vi "查询clonm对应的所有内容.vi"(7 "条件":enum16{"DISTINCT", "MIN", "MAX"}(ring), 8 "error in (no error)":errorcluster caption="错误输入（无错误）", 9 "组合框":string(combo), 10 "database":string="database1.mdb", 11 "table":string(combo)="CODMn") -> (0 "error out":errorcluster caption="错误输出", 3 "输出数组":string[](array[string]))   [LabVIEW 2016]
uses:
  <vilib>/addons/database/Connection.llb/DB Tools Open Connec (String).vi
  <vilib>/addons/database/Connection.llb/Conn Execute.vi
  <vilib>/addons/database/Recordset.llb/Rec Fetch Recordset Data (R).vi
  <vilib>/addons/database/Recordset.llb/Rec Destroy - Connection.vi
  <vilib>/addons/database/_DB Variant To Data/Database Variant To Data.xnode
  <vilib>/addons/database/NI_Database_API.lvlib
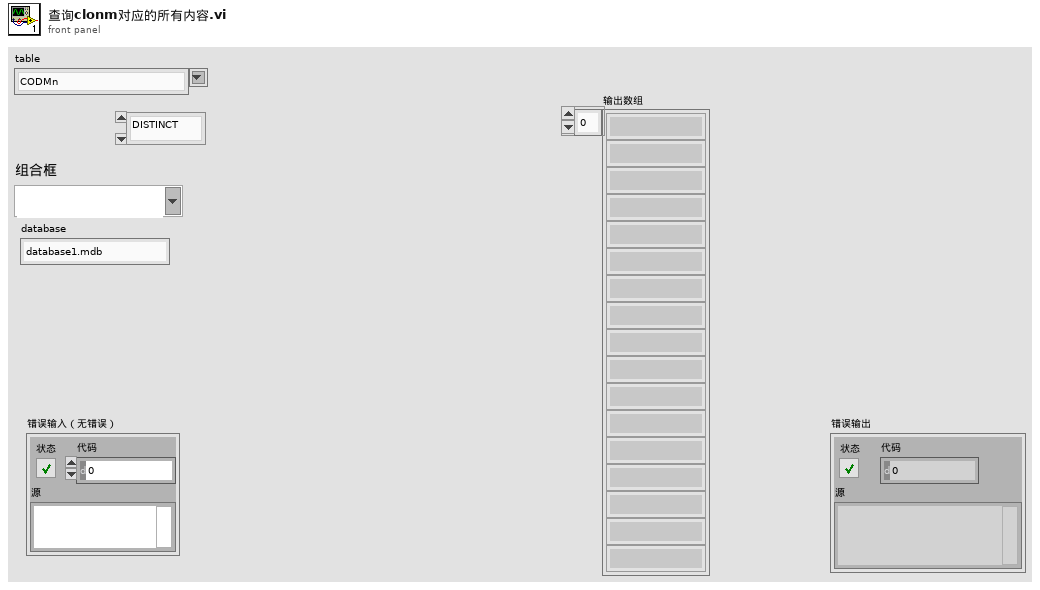
[diagram p1: front panel]
types:
  T1 = typedef "NI_Database_API.lvlib/Conn ObjectReference.ctl" = refnum<k1>
  T2 = typedef "NI_Database_API.lvlib/Rec ObjectReference.ctl" = refnum<k1>
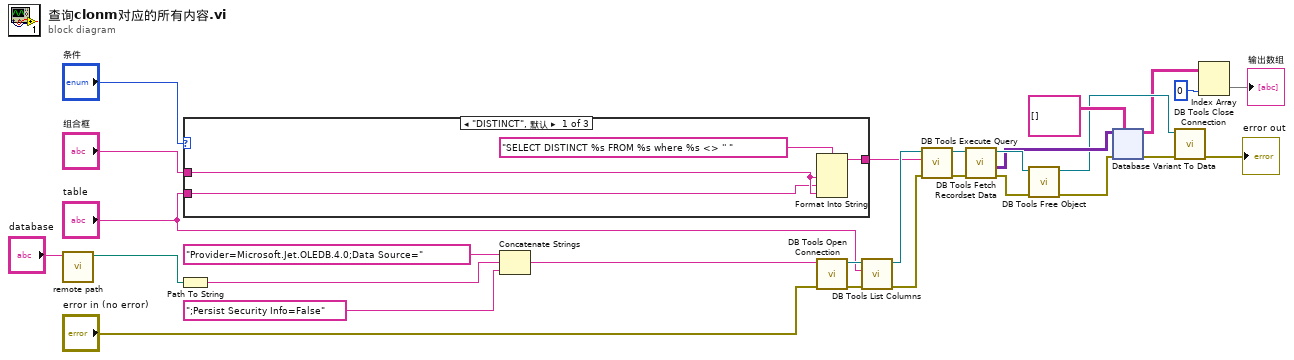
[diagram p0: block diagram]
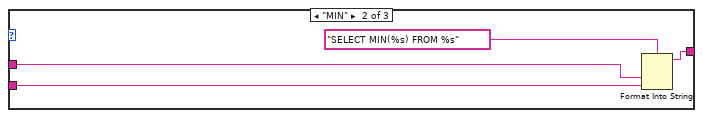
[diagram p2: hidden frame]
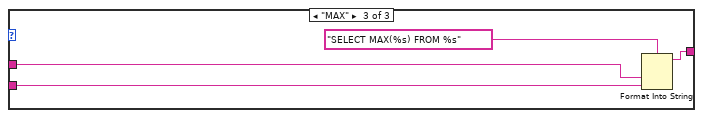
[diagram p3: hidden frame]
diagram:
  n1 = call "remote path.vi"("database"="database") -> ("appended path"=w2:path)  [unwired: 10 in]
  n2 = Path To String(path=w2) -> (string=w24:string)
  n3 = case shown="\"DISTINCT\", 默认" "条件" {
    tunnel: [w32 w33 w37] -> w4
    tunnel: "组合框" -> [w30 w34 w39]
    tunnel: "table" -> [w29 w35 w38]
    frame "DISTINCT", Default {
      n4 = Format Into String(format string="SELECT DISTINCT %s FROM %s where %s <> '' ", w30, w29, w30) -> (resulting string=w32:string)  [unwired: 2 in, 1 out]
    }
    frame "MIN" {
      n5 = Format Into String(format string="SELECT MIN(%s) FROM %s", w34, w35) -> (resulting string=w33:string)  [unwired: 2 in, 1 out]
    }
    frame "MAX" {
      n6 = Format Into String(format string="SELECT MAX(%s) FROM %s", w39, w38) -> (resulting string=w37:string)  [unwired: 2 in, 1 out]
    }
  }
  n7 = Concatenate Strings("Provider=Microsoft.Jet.OLEDB.4.0;Data Source=", w24, ";Persist Security Info=False") -> (w22:string)
  n8 = call-poly <vilib>:"DB Tools Open Connection.vi"("error in (no error)"="error in (no error)", "connection information"=w22) -> ("error out"=w27:errorcluster, "connection reference"=w28:T1)  [unwired: 6 in]
  n9 = call <vilib>:"DB Tools List Columns.vi"("error in (no error)"=w27, "table"="table", "connection reference"=w28) -> ("error out"=w10:errorcluster, "connection reference out"=w11:T1)  [unwired: 1 in, 2 out]
  n10 = call-poly <vilib>:"DB Tools Execute Query.vi"("error in (no error)"=w10, "SQL query"=w4, "connection reference"=w11) -> ("error out"=w20:errorcluster, "recordset reference"=w21:T2)  [unwired: 5 in]
  n11 = call-poly <vilib>:"DB Tools Fetch Recordset Data.vi"("error in (no error)"=w20, "recordset reference"=w21) -> ("error out"=w19:errorcluster, "recordset data"=w15:variant[][], "recordset reference out"=w18:T2)  [unwired: 3 in]
  n12 = call-poly <vilib>:"DB Tools Free Object.vi"("error in (no error)"=w19, "recordset reference"=w18) -> ("error out"=w14:errorcluster, "connection reference"=w13:T1)  [unwired: 8 in]
  n13 = xnode "Database Variant To Data"("database variant"=w15, "error in (no error)"=w14, "type"=string[][] []) -> ("data"=w9:string[][], "error out"=w16:errorcluster)
  n14 = call <vilib>:"DB Tools Close Connection.vi"("error in (no error)"=w16, "connection reference"=w13) -> ("error out"=→"error out":errorcluster)  [unwired: 5 in]
  n15 = Index Array(array=w9, index (col)=0 ("禁用的索引 (列)")) -> (element=→"输出数组":string[])  [unwired: 1 in]
